vi "Cockpit UDP v2.vi"() -> ()   [LabVIEW 2010]
panel:
  out "Waveform Chart 4":sgl(graph)
  out "Waveform Chart 3":sgl(graph)
  out "Waveform Chart 2":sgl(graph)
  out "Waveform Chart":sgl(graph)
  in  "right_pedal":bool
  in  "left_pedal":bool
  in  "up_pedal":bool
  in  "enc 5":sgl
  in  "down_pedal":sgl format="%.2f"
  in  "enc 4":sgl
  in  "enc 3":sgl
  in  "enc 2":sgl
  in  "enc 1":sgl
  in  "stop":bool
  # "Sender"
  # "Receiver"
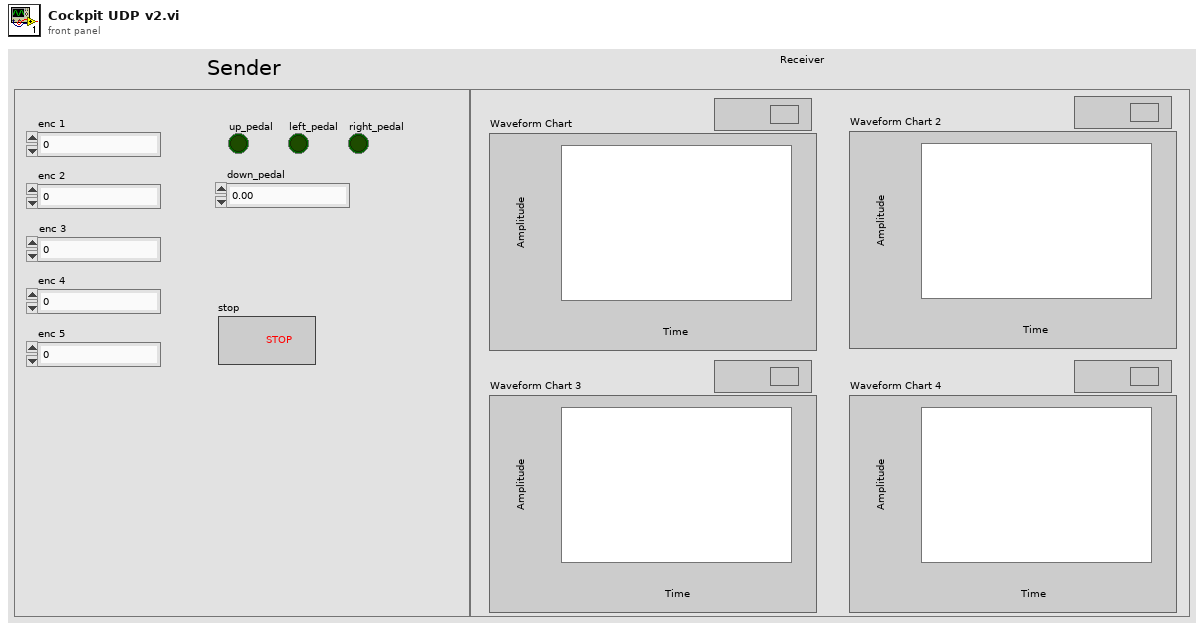
[diagram p1: front panel]
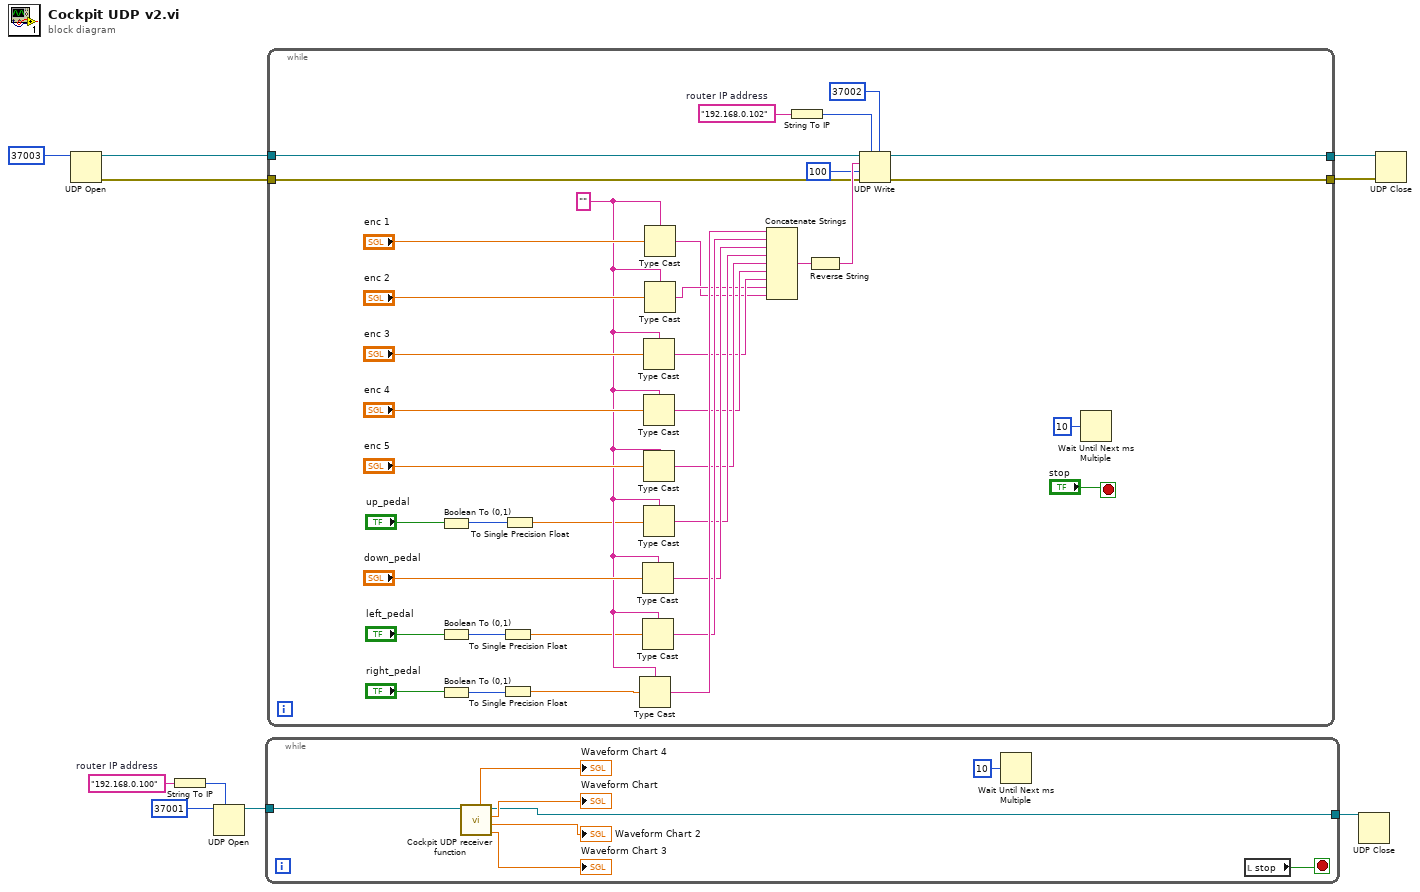
[diagram p0: block diagram]
diagram:
  w4 = "192.168.0.100"  # router IP address
  n1 = UDP Open(11:u16 37003 ("port")) -> (port=w9:refnum<k16>, 0:w7:errorcluster)  [unwired: 4 in, 1 out]
  n2 = String To IP(1:w4) -> (0:w3:u32)
  n3 = UDP Open(7:w3, 11:u16 37001 ("port")) -> (port=w2:refnum<k16>)  [unwired: 3 in, 2 out]
  n4 = while {
    tunnel: w2 -> [w13]
    tunnel: [w12] -> w1
    stop <- w18 stop-if-true
    n5 = call "Cockpit UDP receiver function.vi"("UDP connection ID"=w13) -> ("L3"=→"Waveform Chart 3":sgl, "L2"=→"Waveform Chart 2":sgl, "L1"=→"Waveform Chart":sgl, "UDP connection ID out"=w12:refnum<k16>, "L4"=→"Waveform Chart 4":sgl)  [unwired: 1 in, 5 out]
    n6 = Wait Until Next ms Multiple(millisecond multiple=u32 10) -> ()  [unwired: 1 out]
    n7 = local read "stop"() -> (w18:bool)
  }
  n8 = while {
    tunnel: w9 -> [w49]
    tunnel: [w54] -> w8
    tunnel: w7 -> [w48]
    tunnel: [w53] -> w6
    stop <- "stop" stop-if-true
    w21 = "192.168.0.102"  # router IP address
    w38 = "" ("reversed")
    n9 = Boolean To (0,1)(Boolean="up_pedal") -> (0, 1=w28:i16)
    n10 = Boolean To (0,1)(Boolean="left_pedal") -> (0, 1=w24:i16)
    n11 = Boolean To (0,1)(Boolean="right_pedal") -> (0, 1=w26:i16)
    n12 = To Single Precision Float(number=w24) -> (single precision float=w23:sgl)
    n13 = To Single Precision Float(number=w26) -> (single precision float=w25:sgl)
    n14 = To Single Precision Float(number=w28) -> (single precision float=w27:sgl)
    n15 = Type Cast(type=w38, x=w25) -> (*(type *) &x=w37:string)
    n16 = Type Cast(type=w38, x="down_pedal") -> (*(type *) &x=w35:string)
    n17 = Type Cast(type=w38, x=w23) -> (*(type *) &x=w36:string)
    n18 = Type Cast(type=w38, x="enc 3") -> (*(type *) &x=w31:string)
    n19 = Type Cast(type=w38, x="enc 4") -> (*(type *) &x=w32:string)
    n20 = Type Cast(type=w38, x="enc 5") -> (*(type *) &x=w33:string)
    n21 = Type Cast(type=w38, x=w27) -> (*(type *) &x=w34:string)
    n22 = Type Cast(type=w38, x="enc 1") -> (*(type *) &x=w29:string)
    n23 = Type Cast(type=w38, x="enc 2") -> (*(type *) &x=w30:string)
    n24 = Concatenate Strings(w37, w36, w35, w34, w33, w32, w31, w30, w29) -> (w52:string)
    n25 = String To IP(1:w21) -> (0:w20:u32)
    n26 = Reverse String(1:w52) -> (0:w51:string)
    n27 = UDP Write(address=w20, port or service name=u16 37002, connection ID=w49, data in=w51, 8:w48, 9:100 ("timeout ms (25000)")) -> (error out=w53:errorcluster, 3:w54:refnum<k16>)
    n28 = Wait Until Next ms Multiple(millisecond multiple=u32 10) -> ()  [unwired: 1 out]
  }
  n29 = UDP Close(connection ID=w1) -> ()  [unwired: 1 in, 2 out]
  n30 = UDP Close(connection ID=w8, 8:w6) -> ()  [unwired: 2 out]
